vi "Rotate Thor WP.vi"(3 "error in (no error)":errorcluster, 4 "WP Vals":dbl[](array[numeric])=[0.0, 0.0, 0.0, 0.0, 0.0, 0.0], 5 "input Kcube refnum cluster":T1) -> (0 "error out":errorcluster, 1 "Current Position":sgl[](array[numeric]), 2 "output Kcube cluster":T1)   [LabVIEW 2015]
panel:
  in  "recheck pos time":dbl=0.5 format="%#_13g"
  in  "threshold":dbl=0.1 format="%#_13g"
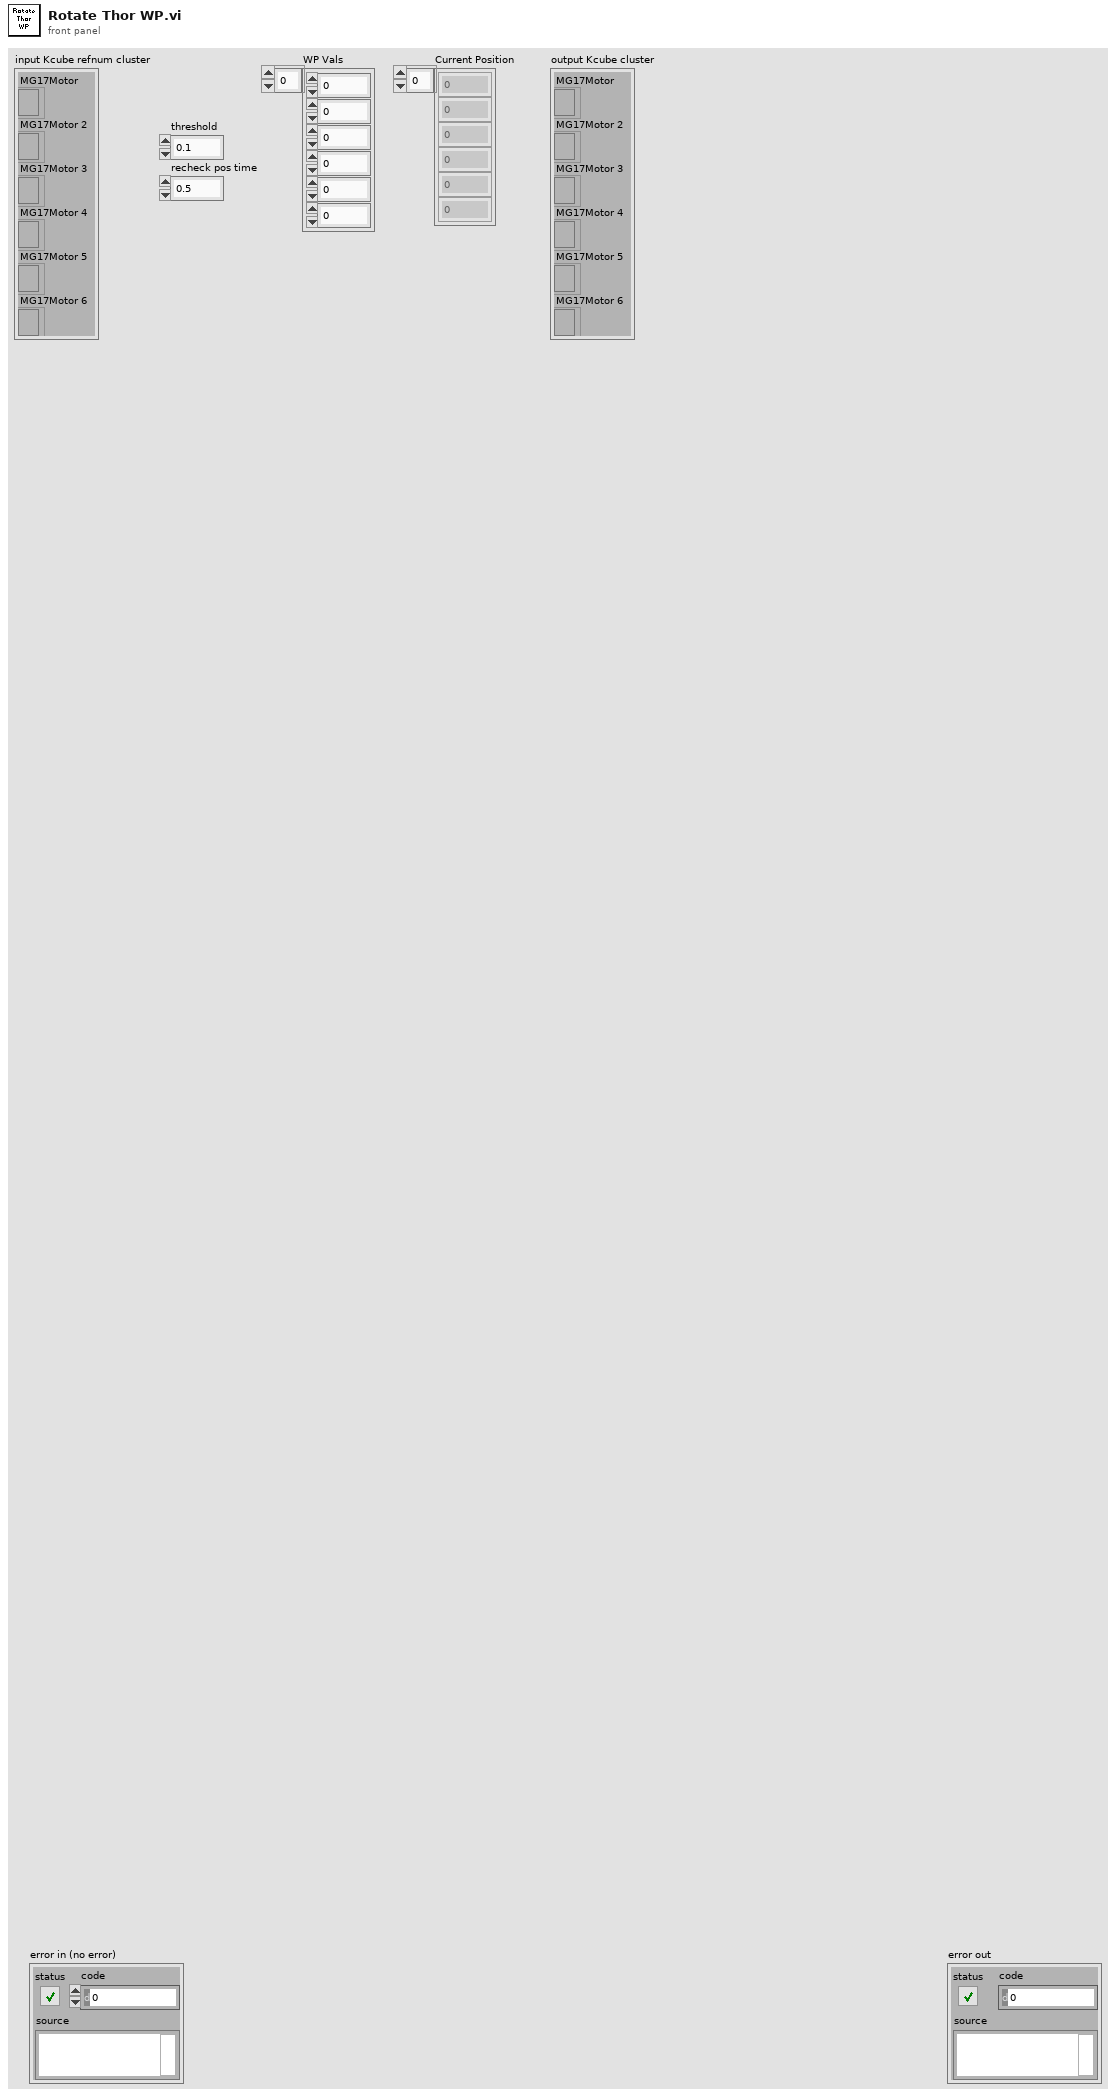
[diagram p1: front panel]
types:
  T1 = cluster{"MG17Motor":refnum<k7>, "MG17Motor 2":refnum<k7>, "MG17Motor 3":refnum<k7>, "MG17Motor 4":refnum<k7>, "MG17Motor 5":refnum<k7>, "MG17Motor 6":refnum<k7>}
  T2 = cluster{"Automation Refnum out":refnum<k7>, "Automation Refnum out":refnum<k7>, "Automation Refnum out":refnum<k7>, "Automation Refnum out":refnum<k7>, "Automation Refnum out":refnum<k7>, "Automation Refnum out":refnum<k7>}
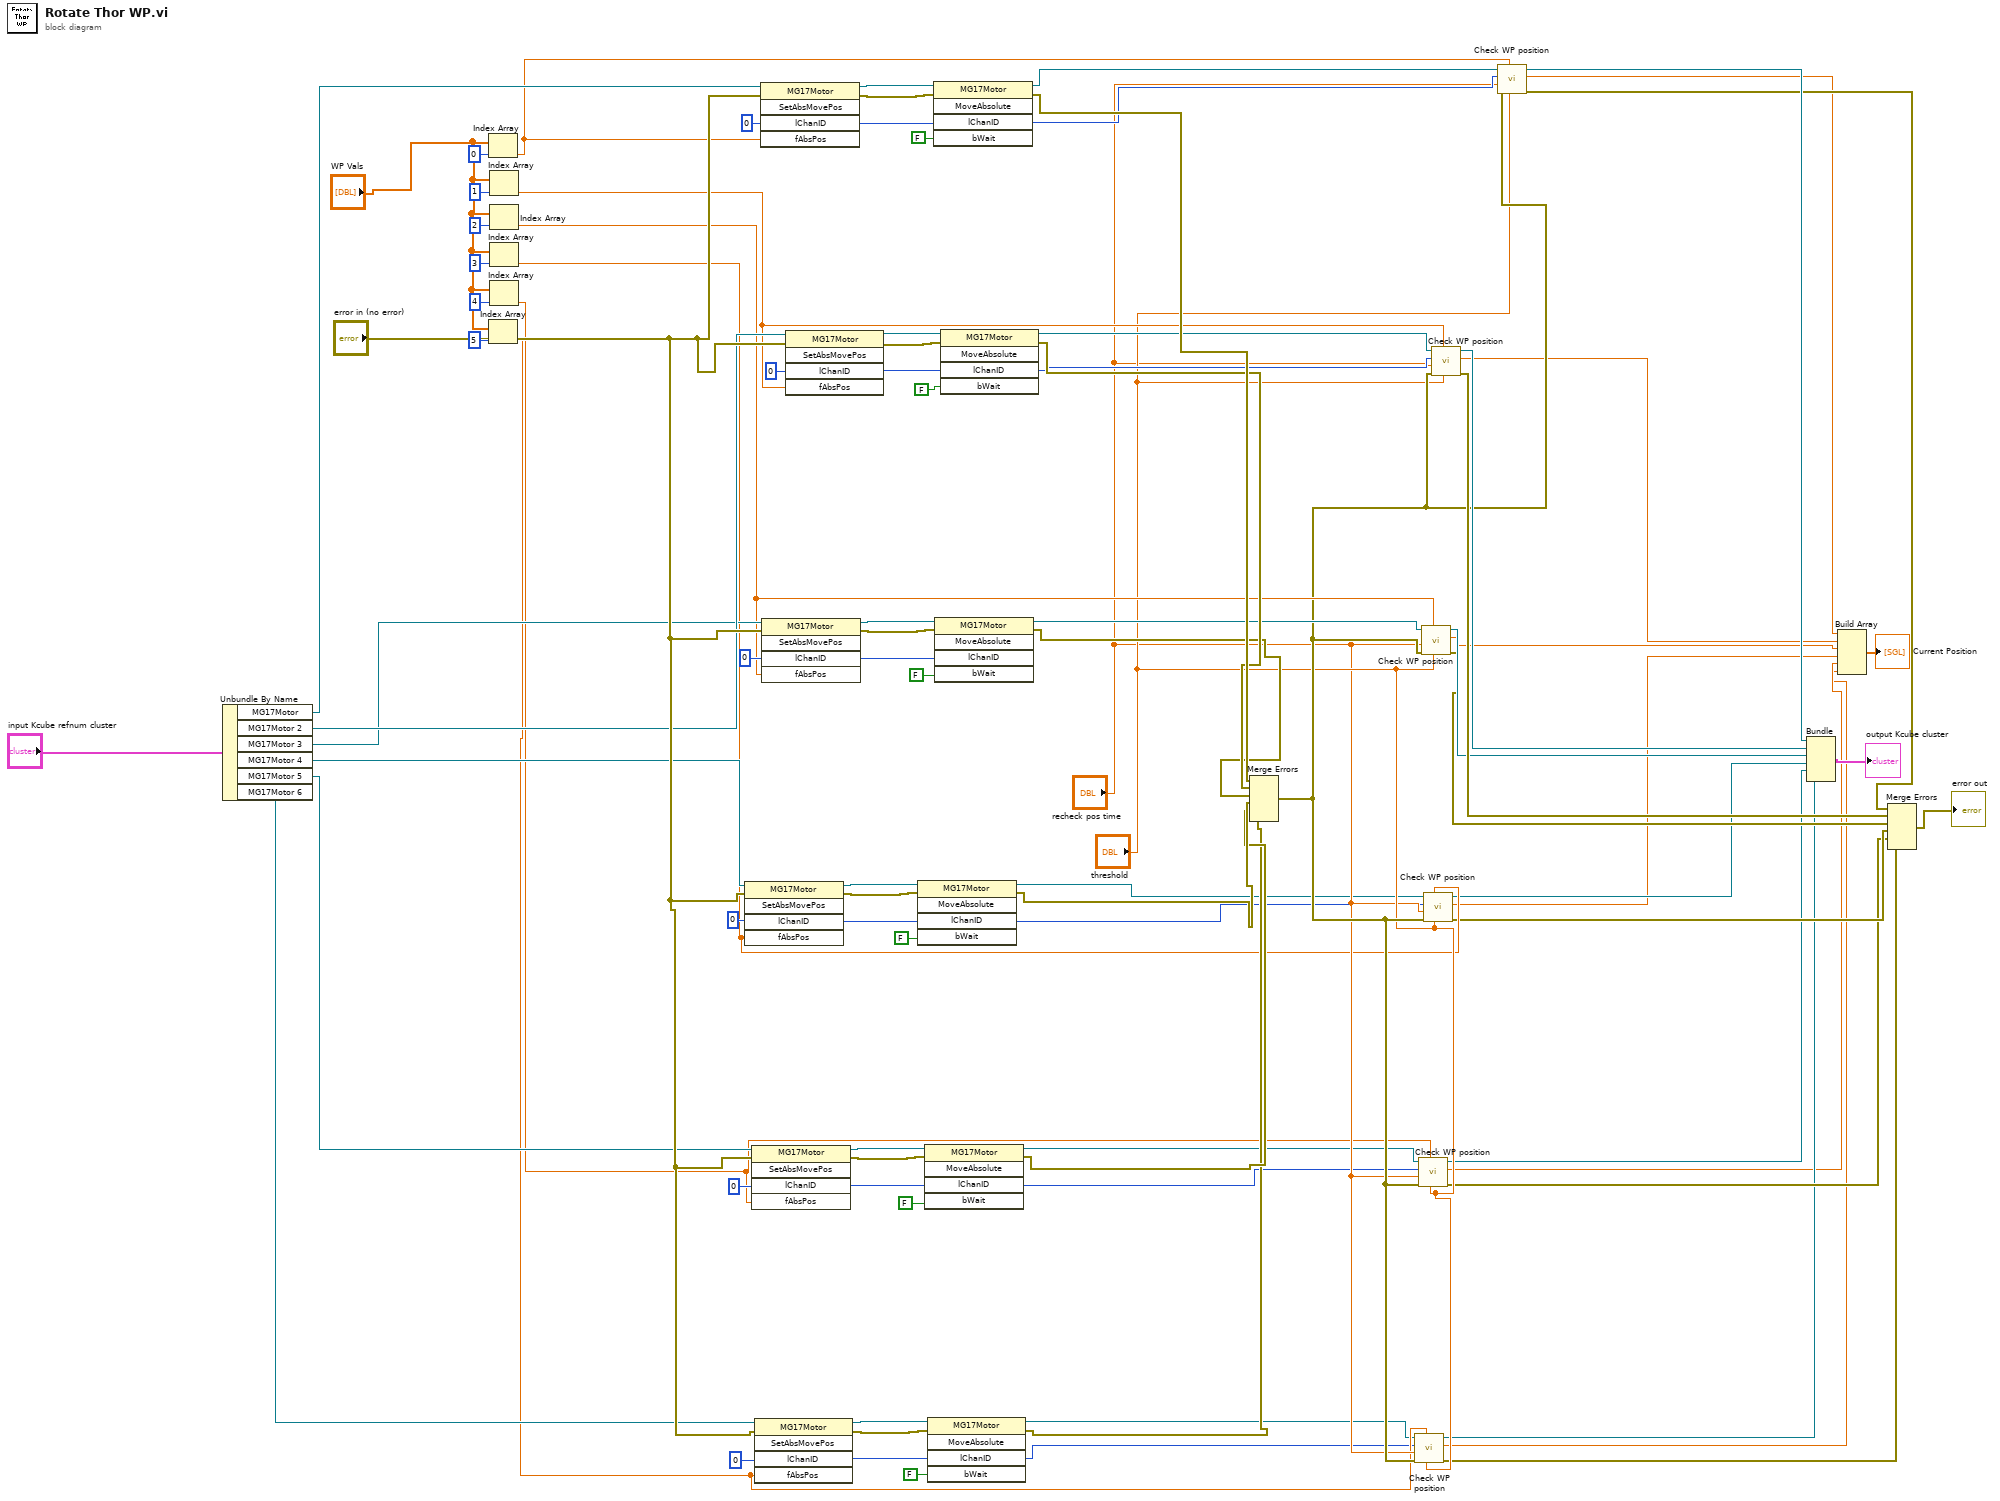
[diagram p0: block diagram]
diagram:
  n1 = Unbundle By Name("input Kcube refnum cluster") -> ("MG17Motor"=w86:refnum<k7>, "MG17Motor 2"=w71:refnum<k7>, "MG17Motor 3"=w70:refnum<k7>, "MG17Motor 4"=w69:refnum<k7>, "MG17Motor 5"=w68:refnum<k7>, "MG17Motor 6"=w67:refnum<k7>)
  n2 = Index Array(array="WP Vals", index=0) -> (element=w38:dbl)
  n3 = Index Array(array="WP Vals", index=5) -> (element=w23:dbl)
  n4 = Index Array(array="WP Vals", index=1) -> (element=w32:dbl)
  n5 = Index Array(array="WP Vals", index=2) -> (element=w29:dbl)
  n6 = Index Array(array="WP Vals", index=3) -> (element=w18:dbl)
  n7 = Index Array(array="WP Vals", index=4) -> (element=w15:dbl)
  n8 = invoke class="MG17Motor" method="SetAbsMovePos"(reference=w69, error in="error in (no error)", "lChanID"=0, "fAbsPos"=w18) -> (reference out=w78:refnum<k7>, error out=w77:errorcluster, "lChanID"=w51:i32)  [unwired: 1 in, 2 out]
  n9 = invoke class="MG17Motor" method="SetAbsMovePos"(reference=w68, error in="error in (no error)", "lChanID"=0, "fAbsPos"=w15) -> (reference out=w76:refnum<k7>, error out=w75:errorcluster, "lChanID"=w50:i32)  [unwired: 1 in, 2 out]
  n10 = invoke class="MG17Motor" method="SetAbsMovePos"(reference=w67, error in="error in (no error)", "lChanID"=0, "fAbsPos"=w23) -> (reference out=w74:refnum<k7>, error out=w73:errorcluster, "lChanID"=w49:i32)  [unwired: 1 in, 2 out]
  n11 = invoke class="MG17Motor" method="SetAbsMovePos"(reference=w86, error in="error in (no error)", "lChanID"=0, "fAbsPos"=w38) -> (reference out=w85:refnum<k7>, error out=w84:errorcluster, "lChanID"=w54:i32)  [unwired: 1 in, 2 out]
  n12 = invoke class="MG17Motor" method="SetAbsMovePos"(reference=w70, error in="error in (no error)", "lChanID"=0, "fAbsPos"=w29) -> (reference out=w80:refnum<k7>, error out=w79:errorcluster, "lChanID"=w52:i32)  [unwired: 1 in, 2 out]
  n13 = invoke class="MG17Motor" method="SetAbsMovePos"(reference=w71, error in="error in (no error)", "lChanID"=0, "fAbsPos"=w32) -> (reference out=w82:refnum<k7>, error out=w81:errorcluster, "lChanID"=w53:i32)  [unwired: 1 in, 2 out]
  n14 = invoke class="MG17Motor" method="MoveAbsolute"(reference=w78, error in=w77, "lChanID"=w51, "bWait"=FALSE) -> (reference out=w20:refnum<k7>, error out=w64:errorcluster, "lChanID"=w19:i32)  [unwired: 1 in, 2 out]
  n15 = invoke class="MG17Motor" method="MoveAbsolute"(reference=w76, error in=w75, "lChanID"=w50, "bWait"=FALSE) -> (reference out=w13:refnum<k7>, error out=w63:errorcluster, "lChanID"=w14:i32)  [unwired: 1 in, 2 out]
  n16 = invoke class="MG17Motor" method="MoveAbsolute"(reference=w74, error in=w73, "lChanID"=w49, "bWait"=FALSE) -> (reference out=w21:refnum<k7>, error out=w62:errorcluster, "lChanID"=w22:i32)  [unwired: 1 in, 2 out]
  n17 = invoke class="MG17Motor" method="MoveAbsolute"(reference=w85, error in=w84, "lChanID"=w54, "bWait"=FALSE) -> (reference out=w41:refnum<k7>, error out=w83:errorcluster, "lChanID"=w39:i32)  [unwired: 1 in, 2 out]
  n18 = invoke class="MG17Motor" method="MoveAbsolute"(reference=w80, error in=w79, "lChanID"=w52, "bWait"=FALSE) -> (reference out=w30:refnum<k7>, error out=w65:errorcluster)  [unwired: 1 in, 3 out]
  n19 = invoke class="MG17Motor" method="MoveAbsolute"(reference=w82, error in=w81, "lChanID"=w53, "bWait"=FALSE) -> (reference out=w34:refnum<k7>, error out=w66:errorcluster, "lChanID"=w33:i32)  [unwired: 1 in, 2 out]
  n20 = Merge Errors(w83, w66, w65, w64, w63, w62) -> (w26:errorcluster)
  n21 = call "Check WP position.vi"("threshold"="threshold", "target"=w23, "error in (no error)"=w26, "recheck pos time"="recheck pos time", "lChanID"=w22, "Automation Refnum in"=w21) -> ("error out"=w10:errorcluster, "Current Position"=w2:sgl, "Automation Refnum out"=w9:refnum<k7>)  [unwired: 3 in]
  n22 = call "Check WP position.vi"("threshold"="threshold", "target"=w15, "error in (no error)"=w26, "recheck pos time"="recheck pos time", "lChanID"=w14, "Automation Refnum in"=w13) -> ("error out"=w11:errorcluster, "Current Position"=w3:sgl, "Automation Refnum out"=w12:refnum<k7>)  [unwired: 3 in]
  n23 = call "Check WP position.vi"("threshold"="threshold", "target"=w29, "error in (no error)"=w26, "recheck pos time"="recheck pos time", "Automation Refnum in"=w30) -> ("error out"=w27:errorcluster, "Current Position"=w5:sgl, "Automation Refnum out"=w28:refnum<k7>)  [unwired: 4 in]
  n24 = call "Check WP position.vi"("threshold"="threshold", "target"=w18, "error in (no error)"=w26, "recheck pos time"="recheck pos time", "lChanID"=w19, "Automation Refnum in"=w20) -> ("error out"=w16:errorcluster, "Current Position"=w4:sgl, "Automation Refnum out"=w17:refnum<k7>)  [unwired: 3 in]
  n25 = call "Check WP position.vi"("threshold"="threshold", "target"=w32, "error in (no error)"=w26, "recheck pos time"="recheck pos time", "lChanID"=w33, "Automation Refnum in"=w34) -> ("error out"=w35:errorcluster, "Current Position"=w6:sgl, "Automation Refnum out"=w31:refnum<k7>)  [unwired: 3 in]
  n26 = call "Check WP position.vi"("threshold"="threshold", "target"=w38, "error in (no error)"=w26, "recheck pos time"="recheck pos time", "lChanID"=w39, "Automation Refnum in"=w41) -> ("error out"=w36:errorcluster, "Current Position"=w7:sgl, "Automation Refnum out"=w40:refnum<k7>)  [unwired: 3 in]
  n27 = Bundle("Automation Refnum out"=w40, "Automation Refnum out"=w31, "Automation Refnum out"=w28, "Automation Refnum out"=w17, "Automation Refnum out"=w12, "Automation Refnum out"=w9) -> (→"output Kcube cluster":T2)  [unwired: 1 in]
  n28 = Build Array(w7, w6, w5, w4, w3, w2) -> (→"Current Position":sgl[])
  n29 = Merge Errors(w36, w35, w27, w16, w11, w10) -> (→"error out":errorcluster)
